vi "Colour Items of a JSON string control.vi"(6 "Defer Panel Updates":bool, 7 "Maximum UI Property calls":i32=-1, 8 "error in (no error)":errorcluster, 10 "String Control":refnum<vi>, 11 "JSON":string) -> (0 "error out":errorcluster)   [LabVIEW 2021, in "jsontext.facade.lvlib"]
doc: "Writes the input JSON to a string control and colour the elements for better readability. Note that this may be slow for large JSON structures; consider the following options\"\n1) Defer Panel Updates set to true will speed up the process by preventing display redraws untill all items are coloured. \n2) You may set a limit to number of elements that are actually coloured in order to ensure the VI completes in a reasonable amount of time (the default of -1 means no limit)."
uses:
  jsontext.facade.lvlib
  jsontext/JSONtext.lvlib
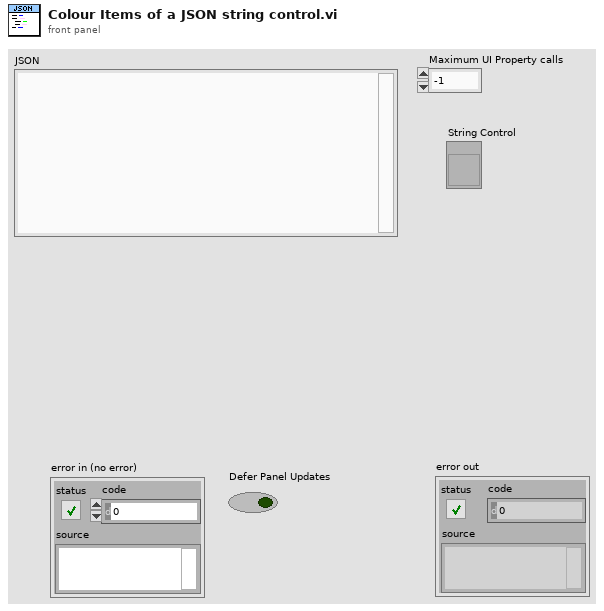
[diagram p1: front panel]
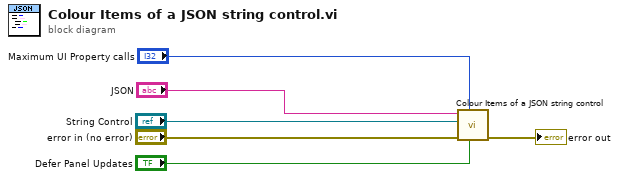
[diagram p0: block diagram]
diagram:
  n1 = call "Colour Items of a JSON string control.vi"("Defer Panel Updates"="Defer Panel Updates", "Maximum UI Property calls"="Maximum UI Property calls", "error in (no error)"="error in (no error)", "String Control"="String Control", "JSON"="JSON") -> ("error out"=→"error out":errorcluster)  [unwired: 6 in]
